vi "Create.vi"(8 "error in (no error)":errorcluster caption="Fehler (Eingang, kein Fehler)", 10 "WhereIGetMyInformationDescription":string, 11 "LoadConfigurationFactory Eingang":refnum<class "LoadConfigurationFactory.lvclass"> caption="DNL_LabVIEW Object in") -> (0 "error out":errorcluster caption="Fehler (Ausgang)", 2 "LoadConfigurationClass.lvclass":refnum<class "LoadConfigurationClass.lvclass">, 3 "LoadConfigurationFactory Ausgang":refnum<class "LoadConfigurationFactory.lvclass"> caption="DNL_LabVIEW Object out")   [LabVIEW 2013, in "LoadConfigurationFactory.lvclass"]
uses:
  LoadConfigurationFactory.lvclass
  LoadConfigurationClass/LoadConfigurationClass.lvclass
  LoadConfigurationFileBasedClass/LoadConfigurationFileBasedClass.lvclass
  LoadConfigurationCsvBasedClass/LoadConfigurationCsvBased.lvclass
panel:
  out "lowercase file extension":string caption="Dateierweiterung in Kleinbuchstaben"
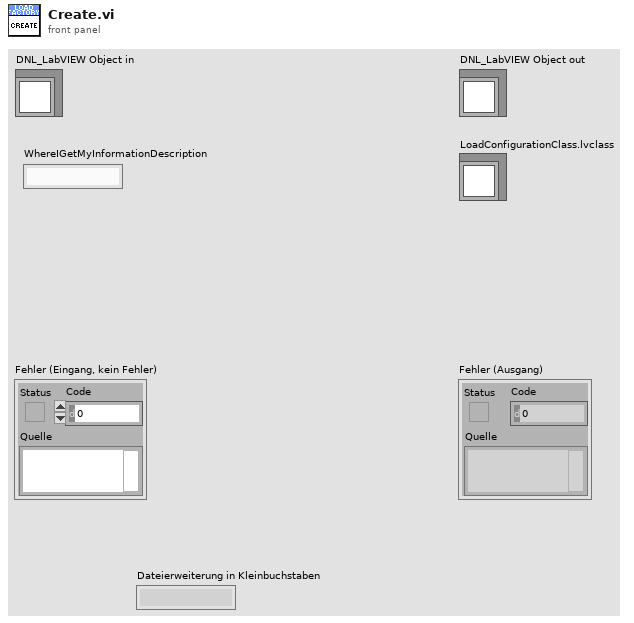
[diagram p1: front panel]
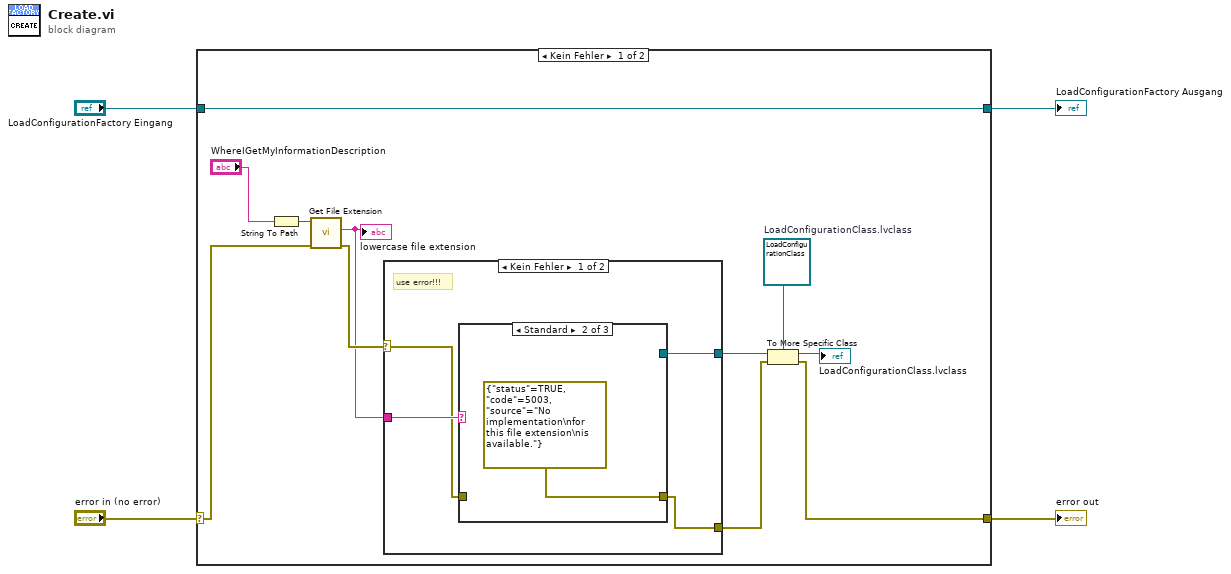
[diagram p0: block diagram]
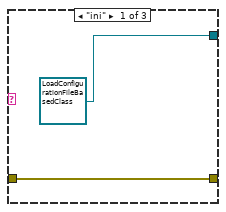
[diagram p2: hidden frame]
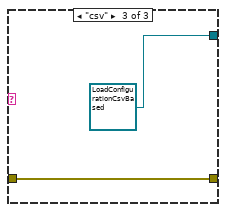
[diagram p3: hidden frame]
diagram:
  n1 = case shown="Kein Fehler" "error in (no error)" {
    selector: "error in (no error)" -> [w12 w27]
    tunnel: [w7 w27] -> w3
    tunnel: [w15 w26] -> w1
    tunnel: "LoadConfigurationFactory Eingang" -> [w15 w26]
    frame No Error {
      w9 = refnum<class "LoadConfigurationClass.lvclass"> refnum  # LoadConfigurationClass.lvclass
      n2 = String To Path(string="WhereIGetMyInformationDescription") -> (path=w14:path)
      n3 = call <vilib>:"Get File Extension.vi"("error in (no error)"=w12, "file"=w14) -> ("error out"=w11:errorcluster, "lowercase file extension"=w10:string)  [unwired: 6 in, 2 out]
      "lowercase file extension" <- w10
      n4 = case shown="Kein Fehler" w11 {
        selector: w11 -> [w17 w25]
        tunnel: w10 -> [w19 _]
        tunnel: [w16 w25] -> w6
        tunnel: [w18 _] -> w5
        frame No Error {
          # "use error!!!"
          n5 = case shown="Standard" w19 {
            tunnel: [refnum<class "LoadConfigurationFileBasedClass.lvclass"> refnum ("LoadConfigurationFileBasedClass.lvclass") _ refnum<class "LoadConfigurationCsvBased.lvclass"> refnum ("LoadConfigurationCsvBased.lvclass")] -> w18
            tunnel: w17 -> [w20 _ w23]
            tunnel: [w20 errorcluster {"status"=TRUE, "code"=5003, "source"="No implementation\nfor this file extension\nis available."} ("error IO") w23] -> w16
            frame "ini" {
            }
            frame Default {
            }
            frame "csv" {
            }
          }
        }
        frame Error {
          # "todo, hier den fehler \ndann reseten"
          # "todo, \n\nmaybe data base connection string"
        }
      }
      n6 = To More Specific Class(target class=w9, reference=w5, error in=w6) -> (specific class reference=→"LoadConfigurationClass.lvclass":refnum<class "LoadConfigurationClass.lvclass">, error out=w7:errorcluster)
    }
    frame Error {
    }
  }
  "error out" <- w3
  "LoadConfigurationFactory Ausgang" <- w1
